vi "Device Init.vi"(8 "错误输入（无错误）":errorcluster caption="Error In(No Error)", 11 "CAN Device In":T1={"Device Type"=20, "Device Index"=0, "CANInd"=0, "Baud(E_U)"=1835016} {"Baud(E_U)" items=["1000Kbps"=393219, "800Kbps"=393220, "500Kbps"=393223, "250Kbps"=1835016, "125Kbps"=1835025, "100Kbps"=1441827, "50Kbps"=1835052, "20Kbps"=1441971, "10Kbps"=1835232, "5Kbps"=1835457]; "Device Type" items=["PCI5121"=1, "PCI9810"=2, "USBCAN1"=3, "USBCAN2"=4, "PCI9820"=5, "PCI5110"=7, "PC104CAN"=11, "CANETUDP"=12, "PCI9840B"=14, "PC104C2"=15, "PCI9820I"=16, "CANETTCP"=17, "PCIE9221"=24, "PCI5010U"=19, "USBCAN_E_U"=20, "USBCAN_2E_U"=21, "PCI5020U"=22, "PCIE9120I"=27, "PCIE9110I"=28, "PCIE9140I"=29, "USBCAN-4E-U"=31, "USBCAN-8E-U"=34]}) -> (0 "错误输出":errorcluster caption="Error Out", 3 "CAN Device Out":T1={"Device Type"=20, "Device Index"=0, "CANInd"=0, "Baud(E_U)"=1835016} {"Baud(E_U)" items=["1000Kbps"=393219, "800Kbps"=393220, "500Kbps"=393223, "250Kbps"=1835016, "125Kbps"=1835025, "100Kbps"=1441827, "50Kbps"=1835052, "20Kbps"=1441971, "10Kbps"=1835232, "5Kbps"=1835457]; "Device Type" items=["PCI5121"=1, "PCI9810"=2, "USBCAN1"=3, "USBCAN2"=4, "PCI9820"=5, "PCI5110"=7, "PC104CAN"=11, "CANETUDP"=12, "PCI9840B"=14, "PC104C2"=15, "PCI9820I"=16, "CANETTCP"=17, "PCIE9221"=24, "PCI5010U"=19, "USBCAN_E_U"=20, "USBCAN_2E_U"=21, "PCI5020U"=22, "PCIE9120I"=27, "PCIE9110I"=28, "PCIE9140I"=29, "USBCAN-4E-U"=31, "USBCAN-8E-U"=34]})   [LabVIEW 2020, in "ZLGCAN.lvclass"]
uses:
  ZLGCAN.lvclass
  Device.ctl
  <vilib>/ErrorRing/Error Ring.xnode
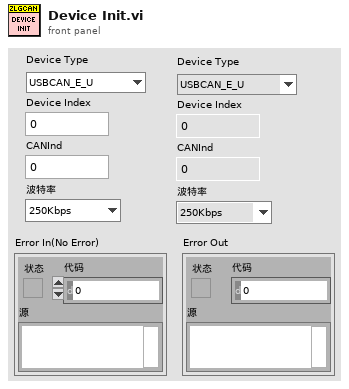
[diagram p1: front panel]
types:
  T1 = typedef "ZLGCAN.lvclass/Device.ctl" = cluster{"Device Type":u32, "Device Index":u32, "CANInd":u32, "Baud(E_U)":u32}
  T2 = cluster{"AccCode":u32, "AccMask":u32, "Reserved":u32, "Filter":u8, "Timing0":u8, "Timing1":u8, "Mode":u8}
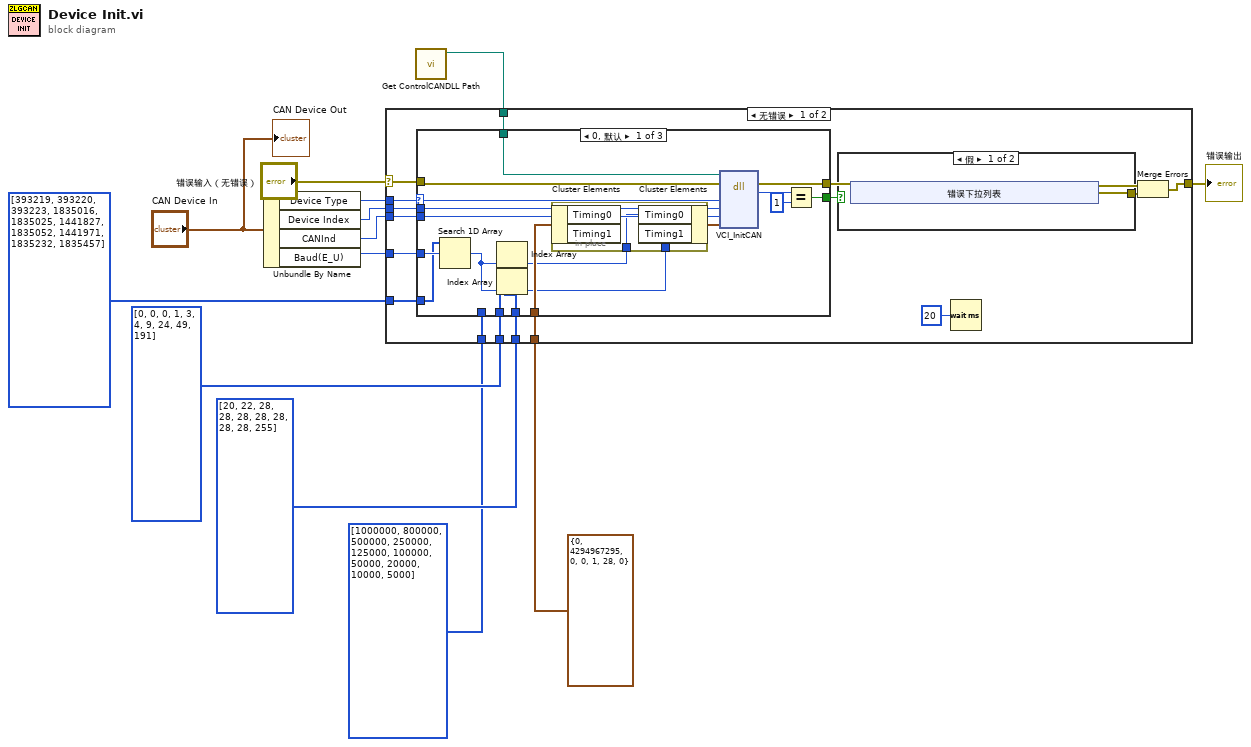
[diagram p0: block diagram]
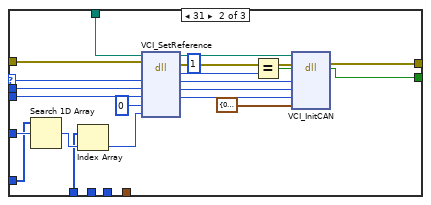
[diagram p2: hidden frame]
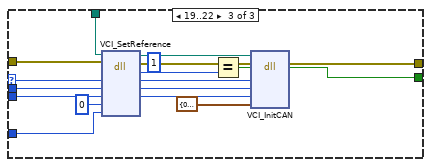
[diagram p3: hidden frame]
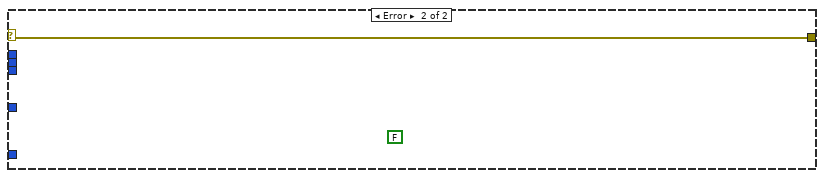
[diagram p5: hidden frame]
diagram:
  n1 = Unbundle By Name("CAN Device In") -> ("Device Type"=w11:u32, "Device Index"=w10:u32, "CANInd"=w9:u32, "Baud(E_U)"=w8:u32)
  n2 = call "Get ControlCANDLL Path.vi"() -> ("拆分的路径"=w1:path)  [unwired: 10 in, 1 out]
  n3 = case shown="无错误" "错误输入（无错误）" {
    selector: "错误输入（无错误）" -> [w22 w90]
    tunnel: [w27 w90] -> w12
    tunnel: w11 -> [w21 _]
    tunnel: w10 -> [w25 _]
    tunnel: w9 -> [w24 _]
    tunnel: w8 -> [w23 _]
    tunnel: u32[] [393219, 393220, 393223, 1835016, 1835025, 1441827, 1835052, 1441971, 1835232, 1835457] ("数组") -> [w20 _]
    tunnel: u8[] [0, 0, 0, 1, 3, 4, 9, 24, 49, 191] ("数组") -> [w19 _]
    tunnel: u8[] [20, 22, 28, 28, 28, 28, 28, 28, 28, 255] ("数组") -> [w18 _]
    tunnel: T2 {"AccCode"=0, "AccMask"=4294967295, "Reserved"=0, "Filter"=0, "Timing0"=1, "Timing1"=28, "Mode"=0} ("VCI_INIT_CONFIG") -> [w16 _]
    tunnel: u32[] [1000000, 800000, 500000, 250000, 125000, 100000, 50000, 20000, 10000, 5000] ("数组") -> [w15 _]
    tunnel: w1 -> [w14 _]
    frame No Error {
      n4 = case shown="0, 默认" w21 {
        selector: w21 -> [w47 w61 w82]
        tunnel: [w40 w58 w87] -> w28
        tunnel: [w43 w62 w80] -> w26
        tunnel: w25 -> [w46 w60 w85]
        tunnel: w24 -> [w45 w59 w84]
        tunnel: w23 -> [w39 w56 w73]
        tunnel: w22 -> [w44 w57 w83]
        tunnel: w20 -> [w38 w55 _]
        tunnel: w19 -> [w37 _ _]
        tunnel: w18 -> [w36 _ _]
        tunnel: w16 -> [w34 _ _]
        tunnel: w15 -> [_ w53 _]
        tunnel: w14 -> [w30 w51 w71]
        frame 0, Default {
          n5 = Search 1D Array(1D array=w38, element=w39) -> (index of element=w35:i32)  [unwired: 1 in]
          n6 = Index Array(array=w37, index=w35) -> (element=w32:u8)
          n7 = Index Array(array=w36, index=w35) -> (element=w31:u8)
          n8 = in-place {
            in-place-border: w32 -> [w49]
            in-place-border: w31 -> [w48]
            n9 = in-place-cluster #1(w34) -> ()  [unwired: 2 out]
            n10 = in-place-cluster #1("Timing0"=w49, "Timing1"=w48) -> (w33:T2)
          }
          n11 = dll-call lib="D:/eDMT Monitor/support/ZLG CAN/ControlCAN.dll" fn="VCI_InitCAN"(path in=w30, error in=w44, "DeviceType"=w47, "DeviceInd"=w46, "CANInd"=w45, "pInitConfig"=w33) -> (error out=w43:errorcluster, "返回类型"=w41:u32)  [unwired: 5 in, 1 out]
          n12 = Equal?(x=w41, y=u32 1) -> (x = y?=w40:bool)
        }
        frame 31 {
          n13 = Search 1D Array(1D array=w55, element=w56) -> (index of element=w54:i32)  [unwired: 1 in]
          n14 = Index Array(array=w53, index=w54) -> (element=w52:u32)
          n15 = dll-call lib="D:/eDMT Monitor/support/ZLG CAN/ControlCAN.dll" fn="VCI_SetReference"(path in=w51, error in=w57, "DevType"=w61, "DevIndex"=w60, "CANInd"=w59, "RefType"=u32 0, "pData"=w52) -> (path out=w50:path, error out=w69:errorcluster, "返回类型"=w63:u32, "DevType"=w67:u32, "DevIndex"=w66:u32, "CANInd"=w65:u32)  [unwired: 3 in]
          n16 = Equal?(x=u32 1 ("y"), y=w63) -> (x = y?=w58:bool)
          n17 = dll-call lib="D:/eDMT Monitor/support/ZLG CAN/ControlCAN.dll" fn="VCI_InitCAN"(path in=w50, error in=w69, "DeviceType"=w67, "DeviceInd"=w66, "CANInd"=w65, "pInitConfig"=T2 {"AccCode"=0, "AccMask"=0, "Reserved"=0, "Filter"=0, "Timing0"=0, "Timing1"=0, "Mode"=0}) -> (error out=w62:errorcluster)  [unwired: 5 in, 2 out]
        }
        frame 19..22 {
          n18 = dll-call lib="D:/eDMT Monitor/support/ZLG CAN/ControlCAN.dll" fn="VCI_SetReference"(path in=w71, error in=w83, "DevType"=w82, "DevIndex"=w85, "CANInd"=w84, "RefType"=u32 0, "pData"=w73) -> (path out=w72:path, error out=w81:errorcluster, "返回类型"=w74:u32, "DevType"=w78:u32, "DevIndex"=w77:u32, "CANInd"=w76:u32)  [unwired: 3 in]
          n19 = Equal?(x=u32 1 ("y"), y=w74) -> (x = y?=w87:bool)
          n20 = dll-call lib="D:/eDMT Monitor/support/ZLG CAN/ControlCAN.dll" fn="VCI_InitCAN"(path in=w72, error in=w81, "DeviceType"=w78, "DeviceInd"=w77, "CANInd"=w76, "pInitConfig"=T2 {"AccCode"=0, "AccMask"=0, "Reserved"=0, "Filter"=0, "Timing0"=0, "Timing1"=0, "Mode"=0}) -> (error out=w80:errorcluster)  [unwired: 5 in, 2 out]
        }
      }
      n21 = case shown="假" w28 {
        tunnel: [w88 _] -> w29
        frame False {
          n22 = xnode "错误下拉列表"() -> ("错误输出"=w88:errorcluster)
        }
        frame True {
        }
      }
      n23 = Wait (ms)(milliseconds to wait=u32 20 ("等待时间（毫秒）")) -> ()  [unwired: 1 out]
      n24 = Merge Errors(w26, w29) -> (w27:errorcluster)
    }
    frame Error {
      (unwired) FALSE
    }
  }
  "错误输出" <- w12
  "CAN Device Out" <- "CAN Device In"
